vi "Connect to Devices.vi"(0 "session in":refnum<k21>, 5 "devices":refnum<k21>="$DefaultDevices", 11 "error in (no error)":errorcluster, 12 "connect timeout (60 sec)":dbl=60.0) -> (4 "session out":refnum<k21>, 15 "error out":errorcluster)   [LabVIEW 2020, in "SLSC.lvlib"]
doc: "Opens network connections for the specified device(s), sharing connections to the same SLSC chassis. For each device that is provided, this VI uses the local configuration file and mDNS to look up the corresponding chassis and its hostname or IP address. If a chassis has multiple hostnames and/or IP addresses, this VI tries connecting using each one, until one succeeds or all have failed. If the connect timeout expires before a connection is successfully established, an error is returned."
uses:
  <vilib>/SLSC/SLSC.lvlib
  nislsclvapi.dll
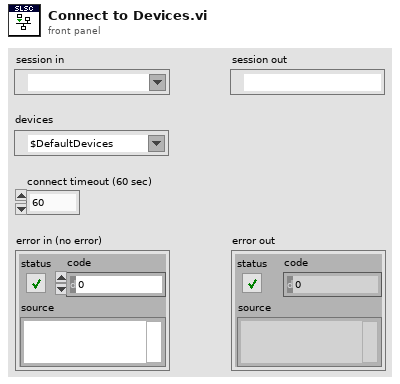
[diagram p1: front panel]
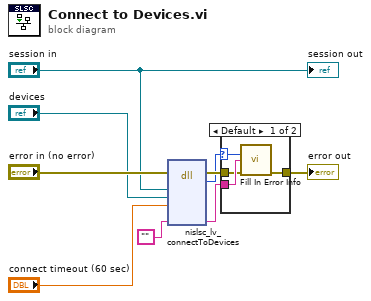
[diagram p0: block diagram]
diagram:
  n1 = dll-call lib="nislsclvapi.*" fn="nislsc_lv_connectToDevices"(error in="error in (no error)", "session"="session in", "devices"="devices", "connectTimeout"="connect timeout (60 sec)", "extendedErrorInfo"="") -> (error out=w6:errorcluster, "return type"=w5:i32, "extendedErrorInfo"=w4:string)  [unwired: 7 in, 1 out]
  n2 = case shown="Default" w5 {
    selector: w5 -> [w13 _]
    tunnel: w4 -> [w12 _]
    tunnel: w6 -> [w11 w14]
    tunnel: [w10 w14] -> w3
    frame Default {
      n3 = call <vilib>:"Fill In Error Info.vi"("status code"=w13, "extended error info"=w12, "error in"=w11) -> ("error out"=w10:errorcluster)  [unwired: 12 in]
    }
    frame 0 {
    }
  }
  "error out" <- w3
  "session out" <- "session in"
